vi "GEA2 Read Message.vi"(0 "GEA2 Event Registration":refnum<event-registration>, 1 "Input Data":T1 {"Command" format="%02x"; "Destination" format="%02x"; "Source" format="%02x"}, 11 "Error In":errorcluster) -> (6 "Raw Data":string, 8 "Coverted Data Out":T2 {"CRC" format="%04x"; "Length" format="%02x"; "Command" format="%02x"; "Destination" format="%02x"; "Source" format="%02x"}, 15 "Error Out":errorcluster)   [LabVIEW 2016, in "GEA2_Toolkit.lvlib"]
doc: "This VI listens on the bus for a specified timeout until the expected command / data is returned."
uses:
  library/GEA2_Toolkit.lvlib
  type defs/Data Out.ctl
  type defs/Data In.ctl
panel:
  out "Command":u8 format="%x"
  out "x = y?":bool
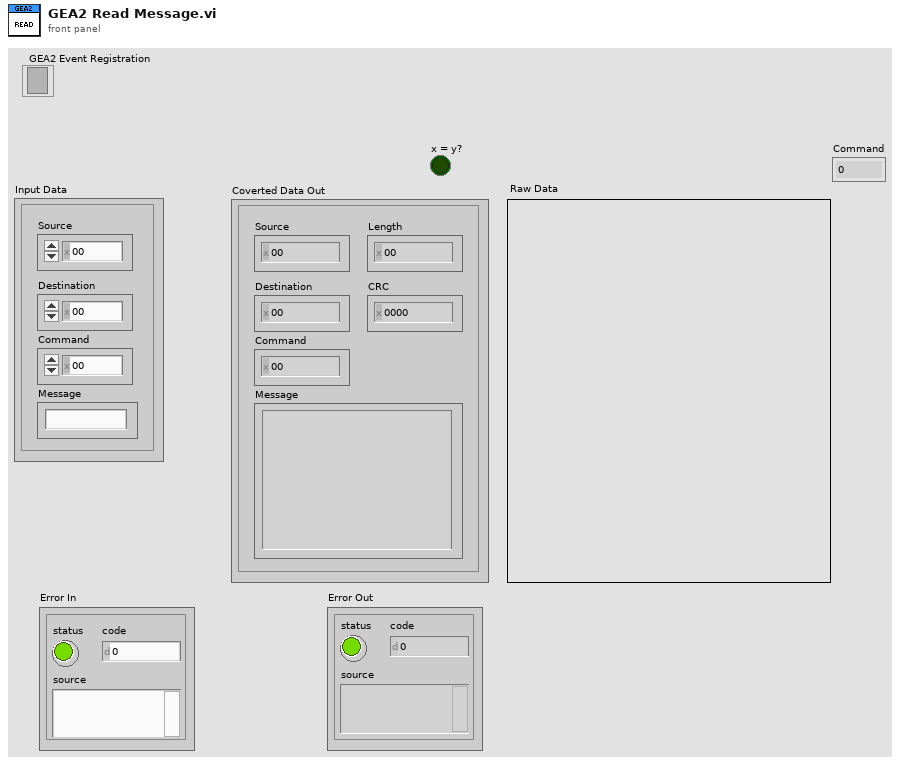
[diagram p1: front panel]
types:
  T1 = typedef "GEA2_Toolkit.lvlib/Data In.ctl" = cluster{"Source":u8, "Destination":u8, "Command":u8, "Message":string}
  T2 = typedef "GEA2_Toolkit.lvlib/Data Out.ctl" = cluster{"Source":u8, "Destination":u8, "Command":u8, "Length":u8, "CRC":u16, "Message":string}
  T3 = typedef "eventsource.ctl" = u32
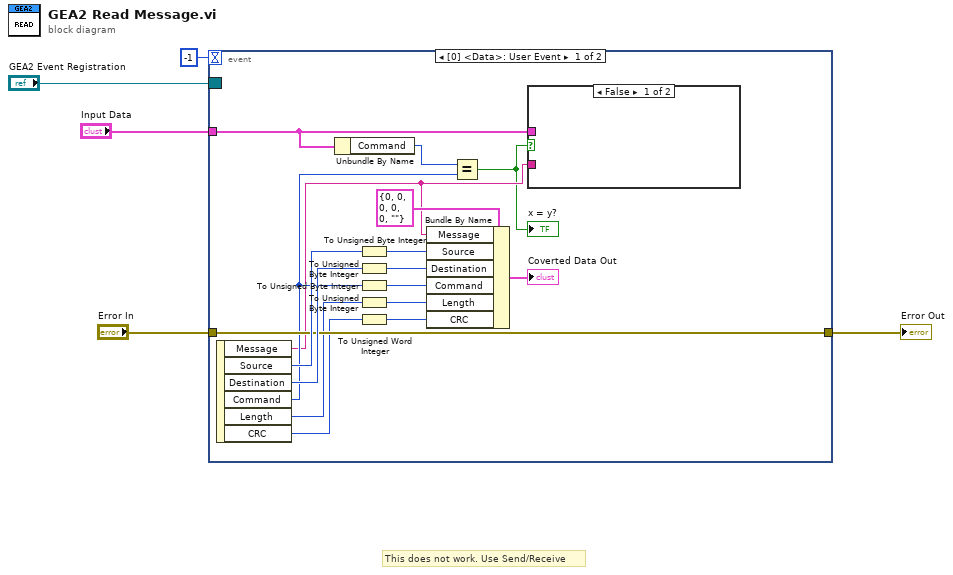
[diagram p0: block diagram]
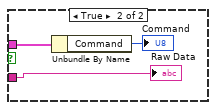
[diagram p2: hidden frame]
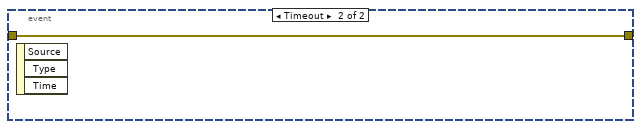
[diagram p3: hidden frame]
diagram:
  # "This does not work. Use Send/Receive"
  n1 = event shown="[0] <Data>: User Event" {
    selector: "GEA2 Event Registration" -> [_ _]
    dyn-events: _ -> [_ _]
    timeout: -1 -> [_ _]
    tunnel: "Error In" -> [w17 w26]
    tunnel: [w17 w26] -> w3
    tunnel: "Input Data" -> [w6 _]
    event User Event {
      n2 = event-data() -> ("Message"=w8:string, "Source"=w18:T3, "Destination"=w19:u8, "Command"=w10:u8, "Length"=w15:u8, "CRC"=w13:u16)  [unwired: 1 in]
      n3 = Unbundle By Name(w6) -> ("Command"=w9:u8)
      n4 = To Unsigned Byte Integer(number=w18) -> (unsigned 8bit integer=w21:u8)
      n5 = To Unsigned Byte Integer(number=w19) -> (unsigned 8bit integer=w22:u8)
      n6 = To Unsigned Byte Integer(number=w10) -> (unsigned 8bit integer=w20:u8)
      n7 = To Unsigned Byte Integer(number=w15) -> (unsigned 8bit integer=w14:u8)
      n8 = To Unsigned Word Integer(number=w13) -> (unsigned 16bit integer=w12:u16)
      n9 = Bundle By Name(cluster=T2 {"Source"=0, "Destination"=0, "Command"=0, "Length"=0, "CRC"=0, "Message"=""} ("Coverted Data Out"), "Message"=w8, "Source"=w21, "Destination"=w22, "Command"=w20, "Length"=w14, "CRC"=w12) -> (→"Coverted Data Out":T2)
      n10 = Equal?(x=w9, y=w10) -> (x = y?=w7:bool)
      "x = y?" <- w7
      n11 = case shown="False" w7 {
        tunnel: w8 -> [_ w23]
        tunnel: w6 -> [_ w25]
        frame False {
        }
        frame True {
          n12 = Unbundle By Name(w25) -> ("Command"=→"Command":u8)
          "Raw Data" <- w23
        }
      }
    }
    event Timeout {
      n13 = event-data() -> ()  [unwired: 1 in, 3 out]
    }
  }
  "Error Out" <- w3
